vi "everything.vi"() -> ()   [LabVIEW 2019]
uses:
  <vilib>/Instr/_visa.llb/VISA Set IO Buffer Mask.ctl
  <vilib>/Instr/_visa.llb/VISA Configure Serial Port (Instr).vi
  <vilib>/express/express shared/transition.llb/Dynamic To Waveform Array.vi
  <vilib>/express/express arith-compare/Formula/Block/exnFormulaBlock how many pts in the wave.vi
  <vilib>/express/express shared/ex_Modify Signal Name.vi
  <vilib>/express/express shared/transition.llb/Waveform Array To Dynamic.vi
  <vilib>/express/express arith-compare/Formula/XNode/ExpressFormulaBlockNode.xnode
panel:
  out "t zone 1":dbl caption="t5"
  out "t supply":dbl caption="t4"
  out "t zone 2":dbl caption="t3"
  out "t zone 3":dbl caption="t6"
  out "t main return":dbl caption="t2"
  out "t inlet":dbl
  out "h zone 1":dbl caption="h5"
  out "h zone 3":dbl caption="h4"
  out "h supply":dbl caption="h4"
  out "h zone 2":dbl caption="h3"
  out "h main return":dbl caption="h2"
  out "h inlet":dbl caption="h1"
  out "c zone 3":dbl caption="zone 3"
  out "c zone 1":dbl caption="zone 1"
  out "c supply":dbl
  out "c zone 2":dbl caption="zone 2"
  out "c main return":dbl caption="main return"
  out "c inlet air":dbl caption="inlet air"
  in  "milliseconds to wait":u32=1000
  out "Voltage 3":dbl format="%.2g"
  out "CFM 3":dbl format="%.2g"
  out "Average CFM 1":dbl format="%.1g"
  out "Voltage 2":dbl format="%#.2g"
  out "CFM 2":dbl format="%.2g"
  out "Average CFM 2":dbl format="%.1g"
  out "CFM 1":dbl format="%.2g"
  out "Average CFM 3":dbl format="%.1g"
  out "Voltage 1":dbl format="%#.2g"
  in  "% Power":dbl min=0.0 max=100.0 step=1.0
  out "Required Voltage":dbl
  in  "Stop":bool
  in  "zone 1 inlet":dbl min=0.0 max=100.0
  in  "zone 1 return":dbl min=0.0 max=100.0
  in  "Fans":i32 min=0 max=1
  in  "zone 2 inlet":dbl min=0.0 max=100.0
  in  "zone 3 inlet":dbl min=0.0 max=100.0
  in  "zone 2 return":dbl min=0.0 max=100.0
  in  "zone 1 co2":dbl min=0.0 max=100.0
  in  "Light 1":i32 min=0 max=1
  in  "fresh air":dbl min=0.0 max=100.0
  in  "zone 2 co2":dbl min=0.0 max=100.0
  in  "Light 3":i32 min=0 max=1
  in  "zone 3 return":dbl min=0.0 max=100.0
  in  "Light 2":i32 min=0 max=1
  in  "zone 3 co2":dbl min=0.0 max=100.0
  in  "VISA- Arduino Uno":refnum<visa-resource-name>
  in  "VISA- Arduino Mega":refnum<visa-resource-name>
  # "Turn off all valves before stopping the VI"
  # "Map for csv Data:\nsupply --> 4\ninlet --> 1\nmain return --> 2\nzone 1--> 5\nzone 2--> 3\nzone 3--> 6"
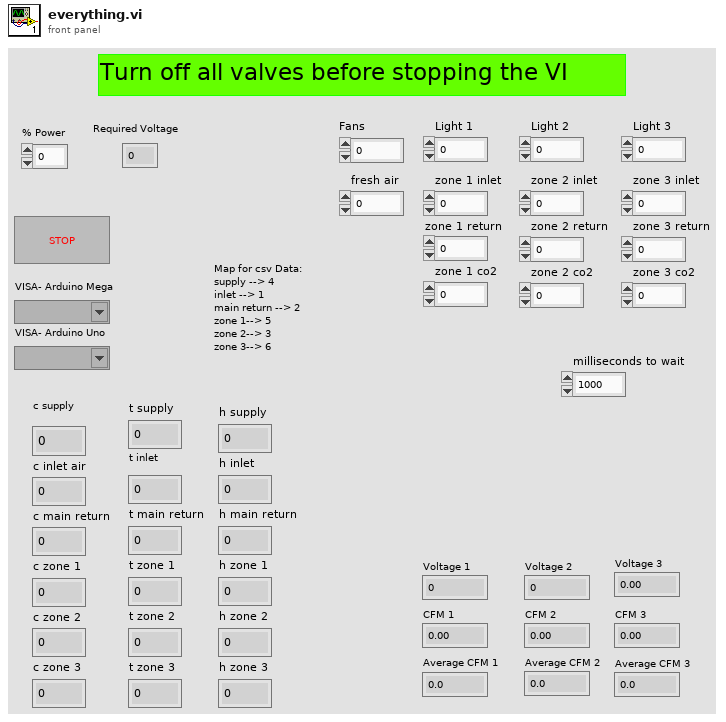
[diagram p1: front panel]
types:
  T1 = typedef "VISA Set IO Buffer Mask.ctl" = u16
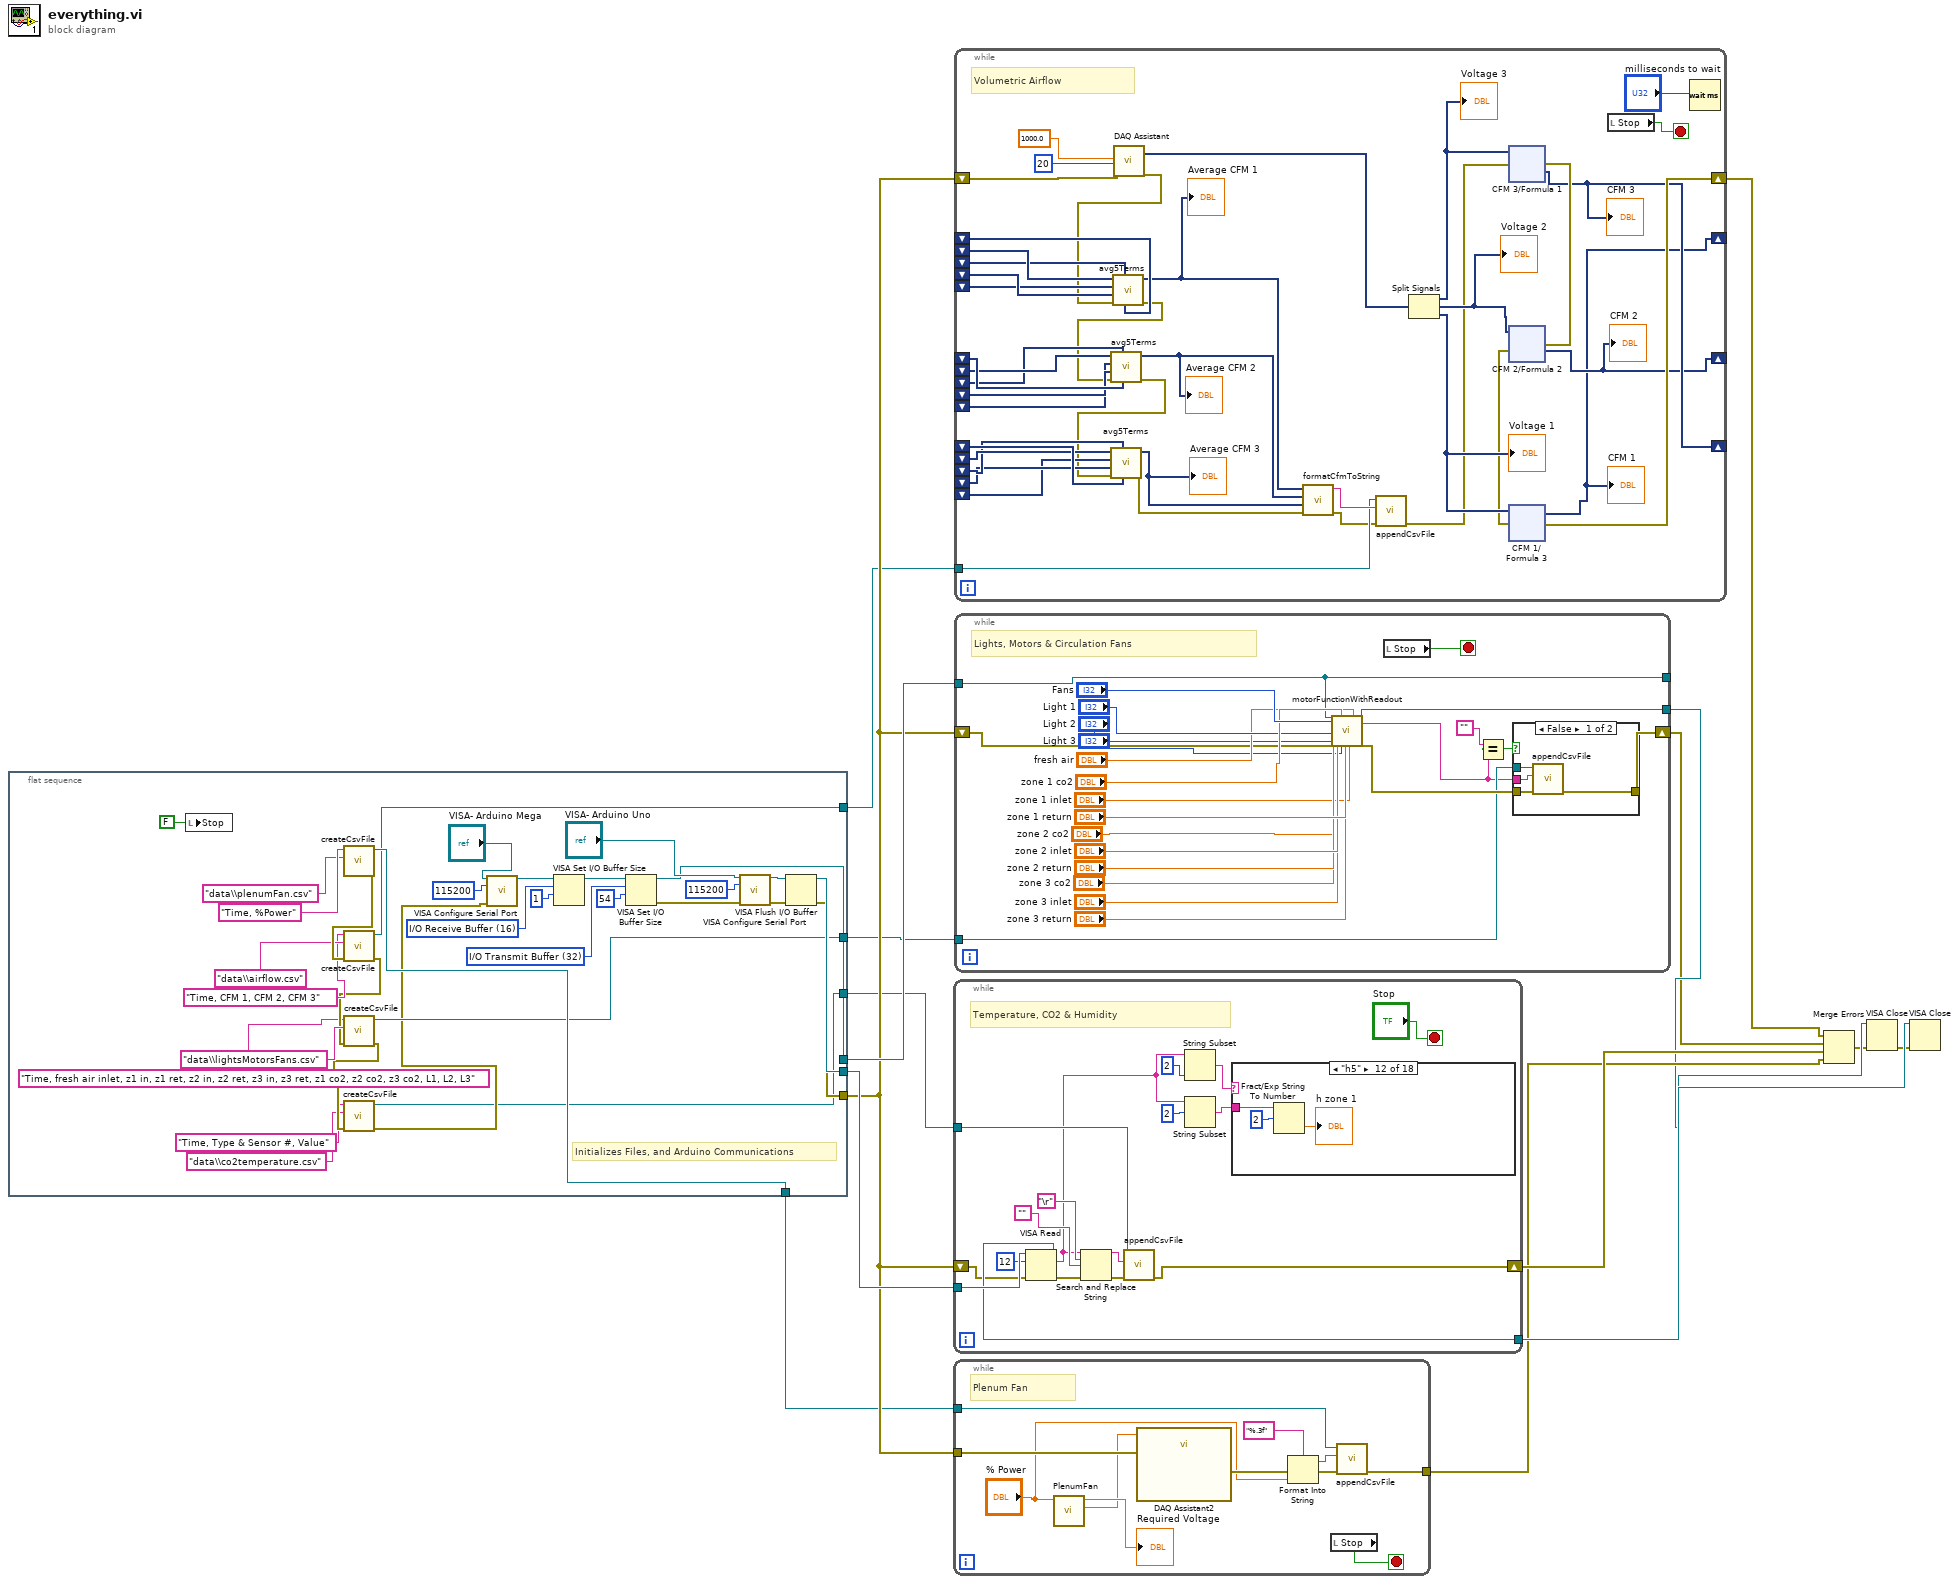
[diagram p0: block diagram]
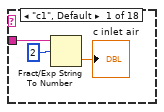
[diagram p2: hidden frame]
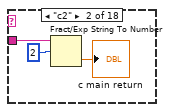
[diagram p3: hidden frame]
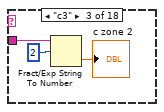
[diagram p4: hidden frame]
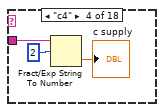
[diagram p5: hidden frame]
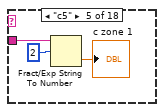
[diagram p6: hidden frame]
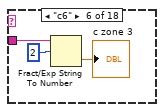
[diagram p7: hidden frame]
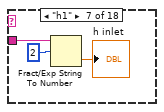
[diagram p8: hidden frame]
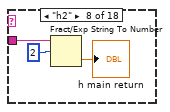
[diagram p9: hidden frame]
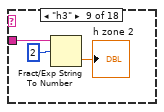
[diagram p10: hidden frame]
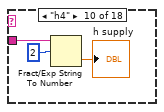
[diagram p11: hidden frame]
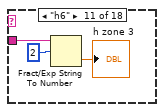
[diagram p12: hidden frame]
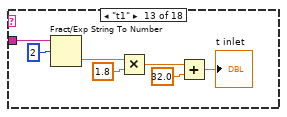
[diagram p13: hidden frame]
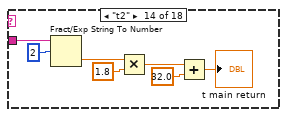
[diagram p14: hidden frame]
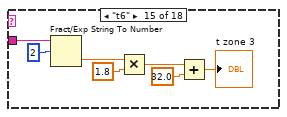
[diagram p15: hidden frame]
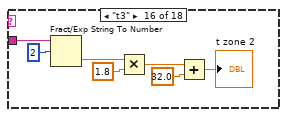
[diagram p16: hidden frame]
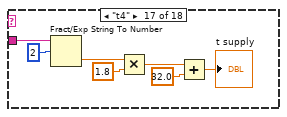
[diagram p17: hidden frame]
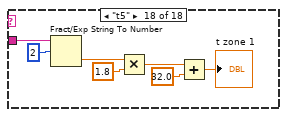
[diagram p18: hidden frame]
diagram:
  n1 = flat-sequence {
    tunnel: [w36] -> w15
    tunnel: [w35] -> w14
    tunnel: [w33] -> w10
    tunnel: [w16] -> w4
    tunnel: [w22] -> w7
    tunnel: [w26] -> w6
    tunnel: [w30] -> w5
    frame #0 {
      w43 = T1 32 items=["I/O Receive Buffer"=16, "I/O Transmit Buffer"=32, "I/O Receive and Transmit Buffer"=48] ("Mask")
      w45 = T1 16 items=["I/O Receive Buffer"=16, "I/O Transmit Buffer"=32, "I/O Receive and Transmit Buffer"=48] ("Mask")
      # "Initializes Files, and Arduino Communications"
      n2 = local write "Stop"(FALSE ("Stop")) -> ()
      n3 = call "createCsvFile.vi"("data\\fileName.csv"="data\\plenumFan.csv" ("replace string (\"\")"), "Header 1, Header 2, etc."="Time, %Power" ("string")) -> ("error out"=w28:errorcluster, "Byte Stream File out"=w30:refnum<file>)  [unwired: 8 in]
      n4 = call "createCsvFile.vi"("error in (no error)"=w28, "data\\fileName.csv"="data\\airflow.csv" ("replace string (\"\")"), "Header 1, Header 2, etc."="Time, CFM 1, CFM 2, CFM 3") -> ("error out"=w23:errorcluster, "Byte Stream File out"=w26:refnum<file>)  [unwired: 7 in]
      n5 = call "createCsvFile.vi"("error in (no error)"=w23, "data\\fileName.csv"="data\\lightsMotorsFans.csv" ("replace string (\"\")"), "Header 1, Header 2, etc."="Time, fresh air inlet, z1 in, z1 ret, z2 in, z2 ret, z3 in, z3 ret, z1 co2, z2 co2, z3 co2, L1, L2, L3") -> ("error out"=w19:errorcluster, "Byte Stream File out"=w22:refnum<file>)  [unwired: 7 in]
      n6 = call "createCsvFile.vi"("error in (no error)"=w19, "data\\fileName.csv"="data\\co2temperature.csv" ("replace string (\"\")"), "Header 1, Header 2, etc."="Time, Type & Sensor #, Value") -> ("error out"=w20:errorcluster, "Byte Stream File out"=w16:refnum<file>)  [unwired: 7 in]
      n7 = call-poly "VISA Configure Serial Port"("VISA resource name"="VISA- Arduino Mega", "baud rate (115200)"=u32 115200 ("baud rate (9600)"), "error in (no error)"=w20) -> ("VISA resource name out"=w47:refnum<visa-resource-name>)  [unwired: 11 in, 1 out]
      n8 = VISA Set I/O Buffer Size(VISA resource name=w47, mask (16)=w45, size (4096)=u32 1) -> (VISA resource name out=w44:refnum<visa-resource-name>)  [unwired: 1 in, 1 out]
      n9 = VISA Set I/O Buffer Size(VISA resource name=w44, mask (16)=w43, size (4096)=u32 54) -> (VISA resource name out=w35:refnum<visa-resource-name>, error out=w34:errorcluster)  [unwired: 1 in]
      n10 = call-poly "VISA Configure Serial Port"("VISA resource name"="VISA- Arduino Uno", "baud rate (115200)"=u32 115200, "error in (no error)"=w34) -> ("VISA resource name out"=w38:refnum<visa-resource-name>, "error out"=w39:errorcluster)  [unwired: 11 in]
      n11 = VISA Flush I/O Buffer(VISA resource name=w38, error in (no error)=w39) -> (VISA resource name out=w36:refnum<visa-resource-name>, error out=w33:errorcluster)  [unwired: 1 in]
    }
  }
  n12 = while {
    shift-right: [w61] -> w12
    shift-left: w10 -> [w63]
    tunnel: w15 -> [w65]
    tunnel: [w64] -> w13
    tunnel: w4 -> [w59]
    stop <- "Stop" stop-if-true
    # "Temperature, CO2 & Humidity"
    n13 = VISA Read(VISA resource name=w65, byte count=u32 12, error in (no error)=w63) -> (VISA resource name out=w64:refnum<visa-resource-name>, read buffer=w49:string, error out=w56:errorcluster)  [unwired: 1 out]
    n14 = Search and Replace String(input string=w49, search string="\r", replace string="", error in=w56) -> (result string=w57:string, error out=w55:errorcluster)  [unwired: 4 in, 2 out]
    n15 = call "appendCsvFile.vi"("error in (no error)"=w55, "text to write"=w57, "Byte Stream File in"=w59) -> ("error out"=w61:errorcluster)  [unwired: 8 in]
    n16 = String Subset(string=w49, length (rest)=2 ("length (rest)")) -> (substring=w52:string)  [unwired: 1 in]
    n17 = String Subset(string=w49, offset (0)=2) -> (substring=w50:string)  [unwired: 1 in]
    n18 = case shown="\"h5\"" w52 {
      tunnel: w50 -> [w67 w70 w73 w76 w79 w82 w85 w88 w91 w94 w97 w100 w107 w114 w121 w128 w135 w142]
      frame "c1", Default {
        n19 = Fract/Exp String To Number(string=w67, offset=2) -> (number=→"c inlet air":dbl)  [unwired: 2 in, 1 out]
      }
      frame "c2" {
        n20 = Fract/Exp String To Number(string=w70, offset=2) -> (number=→"c main return":dbl)  [unwired: 2 in, 1 out]
      }
      frame "c3" {
        n21 = Fract/Exp String To Number(string=w73, offset=2) -> (number=→"c zone 2":dbl)  [unwired: 2 in, 1 out]
      }
      frame "c4" {
        n22 = Fract/Exp String To Number(string=w76, offset=2) -> (number=→"c supply":dbl)  [unwired: 2 in, 1 out]
      }
      frame "c5" {
        n23 = Fract/Exp String To Number(string=w79, offset=2) -> (number=→"c zone 1":dbl)  [unwired: 2 in, 1 out]
      }
      frame "c6" {
        n24 = Fract/Exp String To Number(string=w82, offset=2) -> (number=→"c zone 3":dbl)  [unwired: 2 in, 1 out]
      }
      frame "h1" {
        n25 = Fract/Exp String To Number(string=w85, offset=2) -> (number=→"h inlet":dbl)  [unwired: 2 in, 1 out]
      }
      frame "h2" {
        n26 = Fract/Exp String To Number(string=w88, offset=2) -> (number=→"h main return":dbl)  [unwired: 2 in, 1 out]
      }
      frame "h3" {
        n27 = Fract/Exp String To Number(string=w91, offset=2) -> (number=→"h zone 2":dbl)  [unwired: 2 in, 1 out]
      }
      frame "h4" {
        n28 = Fract/Exp String To Number(string=w94, offset=2) -> (number=→"h supply":dbl)  [unwired: 2 in, 1 out]
      }
      frame "h6" {
        n29 = Fract/Exp String To Number(string=w97, offset=2) -> (number=→"h zone 3":dbl)  [unwired: 2 in, 1 out]
      }
      frame "h5" {
        n30 = Fract/Exp String To Number(string=w100, offset=2) -> (number=→"h zone 1":dbl)  [unwired: 2 in, 1 out]
      }
      frame "t1" {
        n31 = Fract/Exp String To Number(string=w107, offset=2) -> (number=w106:dbl)  [unwired: 2 in, 1 out]
        n32 = Multiply(x=w106, y=1.8) -> (x*y=w104:dbl)
        n33 = Add(x=w104, y=32.0) -> (x+y=→"t inlet":dbl)
      }
      frame "t2" {
        n34 = Fract/Exp String To Number(string=w114, offset=2) -> (number=w113:dbl)  [unwired: 2 in, 1 out]
        n35 = Multiply(x=w113, y=1.8) -> (x*y=w111:dbl)
        n36 = Add(x=w111, y=32.0) -> (x+y=→"t main return":dbl)
      }
      frame "t6" {
        n37 = Fract/Exp String To Number(string=w121, offset=2) -> (number=w120:dbl)  [unwired: 2 in, 1 out]
        n38 = Multiply(x=w120, y=1.8) -> (x*y=w118:dbl)
        n39 = Add(x=w118, y=32.0) -> (x+y=→"t zone 3":dbl)
      }
      frame "t3" {
        n40 = Fract/Exp String To Number(string=w128, offset=2) -> (number=w127:dbl)  [unwired: 2 in, 1 out]
        n41 = Multiply(x=w127, y=1.8) -> (x*y=w125:dbl)
        n42 = Add(x=w125, y=32.0) -> (x+y=→"t zone 2":dbl)
      }
      frame "t4" {
        n43 = Fract/Exp String To Number(string=w135, offset=2) -> (number=w134:dbl)  [unwired: 2 in, 1 out]
        n44 = Multiply(x=w134, y=1.8) -> (x*y=w132:dbl)
        n45 = Add(x=w132, y=32.0) -> (x+y=→"t supply":dbl)
      }
      frame "t5" {
        n46 = Fract/Exp String To Number(string=w142, offset=2) -> (number=w141:dbl)  [unwired: 2 in, 1 out]
        n47 = Multiply(x=w141, y=1.8) -> (x*y=w139:dbl)
        n48 = Add(x=w139, y=32.0) -> (x+y=→"t zone 1":dbl)
      }
    }
  }
  n49 = while {
    tunnel: [w147] -> w11
    tunnel: w10 -> [w153]
    tunnel: w5 -> [w145]
    stop <- w152 stop-if-true
    # "Plenum Fan"
    n50 = call "PlenumFan.vi"("% Power"="% Power") -> ("Numeric"=w151:dbl, "Required Voltage"=→"Required Voltage":dbl)  [unwired: 9 in]
    n51 = call "DAQ Assistant2"("data"=w151, "error in"=w153) -> ("error out"=w149:errorcluster)  [unwired: 16 in, 1 out]
    n52 = Format Into String(format string="%.3f", error in=w149, "% Power") -> (resulting string=w146:string, error out=w148:errorcluster)  [unwired: 1 in]
    n53 = local read "Stop"() -> (w152:bool)
    n54 = call "appendCsvFile.vi"("error in (no error)"=w148, "text to write"=w146, "Byte Stream File in"=w145) -> ("error out"=w147:errorcluster)  [unwired: 8 in]
  }
  n55 = while {
    shift-right: [w156] -> _
    shift-left: _ -> [w175]
    shift-left: _ -> [w172]
    shift-left: _ -> [w173]
    shift-right: [w157] -> _
    shift-left: _ -> [w180]
    shift-left: _ -> [w178]
    shift-left: _ -> [w177]
    shift-left: _ -> [w174]
    shift-left: _ -> [w171]
    shift-left: _ -> [w179]
    shift-left: _ -> [w176]
    shift-right: [w158] -> _
    shift-left: _ -> [w185]
    shift-left: _ -> [w184]
    shift-left: _ -> [w183]
    shift-left: _ -> [w182]
    shift-left: _ -> [w181]
    shift-right: [w189] -> w9
    shift-left: w10 -> [w188]
    tunnel: w6 -> [w161]
    stop <- w168 stop-if-true
    # "Volumetric Airflow"
    n56 = call "DAQ Assistant"("rate"=1000.0, "number of samples"=20, "error in"=w188) -> ("data"=w195:dynamicdata, "error out"=w170:errorcluster)  [unwired: 14 in, 1 out]
    n57 = call "avg5Terms.vi"("Result"=w175, "Result 3"=w173, "error in (no error)"=w170, "Result 4"=w172, "Result 5"=w171, "Result 2"=w174) -> ("error out"=w169:errorcluster, "Dynamic Data"=w163:dynamicdata)  [unwired: 4 in]
    "Average CFM 1" <- w163
    n58 = call "avg5Terms.vi"("Result"=w180, "Result 3"=w178, "error in (no error)"=w169, "Result 4"=w177, "Result 5"=w176, "Result 2"=w179) -> ("error out"=w167:errorcluster, "Dynamic Data"=w164:dynamicdata)  [unwired: 4 in]
    "Average CFM 2" <- w164
    n59 = call "avg5Terms.vi"("Result"=w185, "Result 3"=w183, "error in (no error)"=w167, "Result 4"=w182, "Result 5"=w181, "Result 2"=w184) -> ("error out"=w166:errorcluster, "Dynamic Data"=w165:dynamicdata)  [unwired: 4 in]
    "Average CFM 3" <- w165
    n60 = call "formatCfmToString.vi"("error in (no error)"=w166, "CFM 1"=w165, "CFM 2"=w164, "CFM 3"=w163) -> ("error out"=w160:errorcluster, "String"=w162:string)  [unwired: 6 in]
    n61 = call "appendCsvFile.vi"("error in (no error)"=w160, "text to write"=w162, "Byte Stream File in"=w161) -> ("error out"=w159:errorcluster)  [unwired: 8 in]
    n62 = Split Signals(w195) -> (w192:dynamicdata, w193:dynamicdata, w194:dynamicdata)  [unwired: 3 in]
    "Voltage 3" <- w192
    "Voltage 2" <- w193
    "Voltage 1" <- w194
    n63 = xnode "CFM 3/Formula 1"("X1"=w192, "error in (no error)"=w159) -> ("Result"=w158:dynamicdata, "error out"=w191:errorcluster)
    "CFM 3" <- w158
    n64 = xnode "CFM 2/Formula 2"("X1"=w193, "error in (no error)"=w191) -> ("Result"=w157:dynamicdata, "error out"=w190:errorcluster)
    "CFM 2" <- w157
    n65 = xnode "CFM 1/\nFormula 3"("X1"=w194, "error in (no error)"=w190) -> ("Result"=w156:dynamicdata, "error out"=w189:errorcluster)
    "CFM 1" <- w156
    n66 = local read "Stop"() -> (w168:bool)
    n67 = Wait (ms)(milliseconds to wait="milliseconds to wait") -> ()  [unwired: 1 out]
  }
  n68 = while {
    shift-right: [w616] -> w1
    shift-left: w10 -> [w623]
    tunnel: w14 -> [w613]
    tunnel: [w622] -> w8
    tunnel: w7 -> [w617]
    tunnel: [w613] -> _
    stop <- w620 stop-if-true
    # "Lights, Motors & Circulation Fans"
    n69 = call "motorFunctionWithReadout.vi"("VISA Refnum in"=w613, "Fans"="Fans", "zone 3 co2"="zone 3 co2", "zone 2 return"="zone 2 return", "Light 1"="Light 1", "zone 2 co2"="zone 2 co2", "Light 3"="Light 3", "error in (no error)"=w623, "zone 2 inlet"="zone 2 inlet", "zone 3 inlet"="zone 3 inlet", "zone 1 co2"="zone 1 co2", "Light 2"="Light 2", "zone 1 return"="zone 1 return", "zone 3 return"="zone 3 return", "zone 1 inlet"="zone 1 inlet", "fresh air"="fresh air") -> ("String"=w615:string, "VISA Refnum out"=w622:refnum<visa-resource-name>, "error out"=w618:errorcluster)  [unwired: 9 in]
    n70 = local read "Stop"() -> (w620:bool)
    n71 = Equal?(x="", y=w615) -> (x = y?=w619:bool)
    n72 = case shown="False" w619 {
      tunnel: w618 -> [w640 w641]
      tunnel: w617 -> [w639 _]
      tunnel: [w638 w641] -> w616
      tunnel: w615 -> [w637 _]
      frame False {
        n73 = call "appendCsvFile.vi"("error in (no error)"=w640, "text to write"=w637, "Byte Stream File in"=w639) -> ("error out"=w638:errorcluster)  [unwired: 8 in]
      }
      frame True {
      }
    }
  }
  n74 = Merge Errors(w9, w1, w12, w11) -> (w2:errorcluster)
  n75 = VISA Close(VISA resource name=w8, error in (no error)=w2) -> (error out=w3:errorcluster)
  n76 = VISA Close(VISA resource name=w13, error in (no error)=w3) -> ()  [unwired: 1 out]
